vi "WaitOnSocketListener.vi"(0 "Universal Robot.lvclass in":refnum<class "Universal Robot.lvclass">, 2 "Timeout (ms)":i32, 5 "error in (no error)":errorcluster) -> (14 "Universal Robot.lvclass out":refnum<class "Universal Robot.lvclass">, 19 "error out":errorcluster)   [LabVIEW 2019, in "Universal Robot.lvclass"]
uses:
  Universal Robot.lvclass
  Universal Robot.lvclass/Universal Robot.ctl
  Client Interfaces/Socket Communication/Socket Communication.lvclass
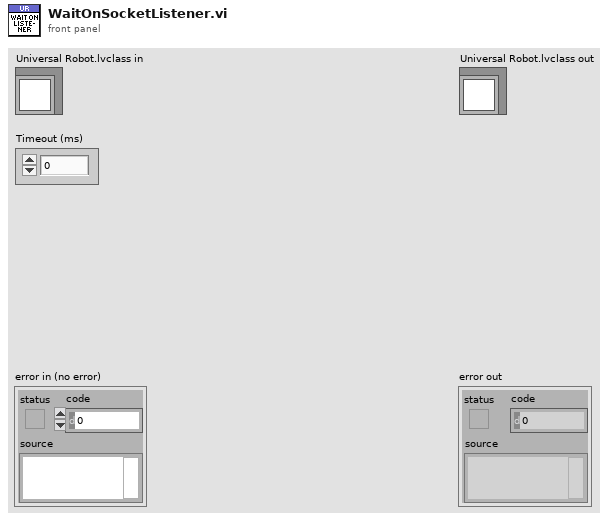
[diagram p1: front panel]
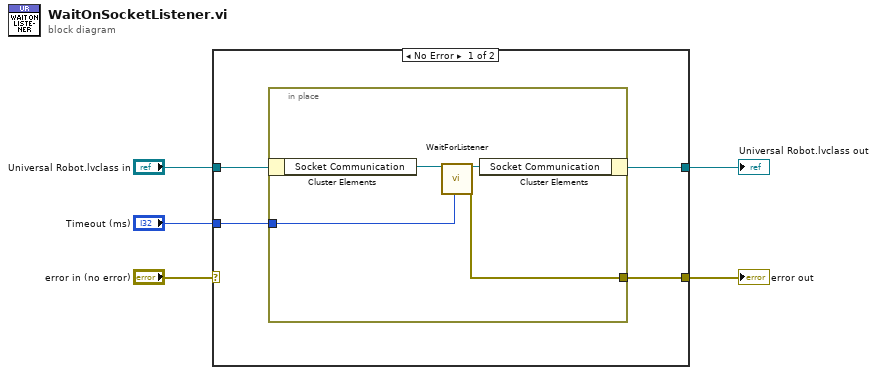
[diagram p0: block diagram]
diagram:
  n1 = case shown="No Error" "error in (no error)" {
    selector: "error in (no error)" -> [_ w15]
    tunnel: [w9 w15] -> w4
    tunnel: "Universal Robot.lvclass in" -> [w8 w14]
    tunnel: [w7 w14] -> w2
    tunnel: "Timeout (ms)" -> [w6 _]
    frame No Error {
      n2 = in-place {
        in-place-border: [w11] -> w9
        in-place-border: w6 -> [w10]
        n3 = in-place-cluster #1(w8) -> ("Socket Communication"=w13:refnum<class "Socket Communication.lvclass">)
        n4 = call "WaitForListener.vi"("Socket Listener in"=w13, "Timeout (ms)"=w10) -> ("Socket Listener out"=w12:refnum<class "Socket Communication.lvclass">, "error out"=w11:errorcluster)  [unwired: 16 in]
        n5 = in-place-cluster #1("Socket Communication"=w12) -> (w7:refnum<class "Universal Robot.lvclass">)
      }
    }
    frame Error {
    }
  }
  "error out" <- w4
  "Universal Robot.lvclass out" <- w2
